vi "Write Assert VI UID.vi"(10 "Assert VI UID":i32, 11 "Show Assert in":refnum<class "Show Assert.lvclass">) -> (3 "Show Assert out":refnum<class "Show Assert.lvclass">)   [LabVIEW 2016, in "Assert API Components.lvlib" / "Assert Display.lvlib" / "Main Display.lvlib" / "Show Assert.lvclass"]
uses:
  Show Assert.lvclass
  Show Assert.lvclass/Show Assert.ctl
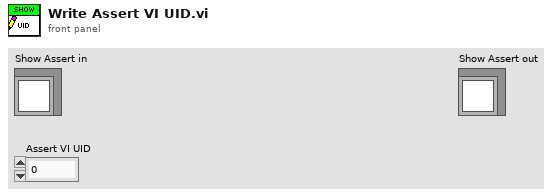
[diagram p1: front panel]
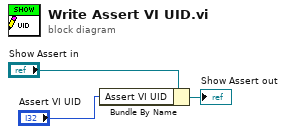
[diagram p0: block diagram]
diagram:
  n1 = Bundle By Name(cluster="Show Assert in", "Assert VI UID"="Assert VI UID") -> (→"Show Assert out":refnum<class "Show Assert.lvclass">)
